vi "First model found in list.vi"(8 "Models to look for":string[](array[string])=["33120A", "33220A", "AFG2021"], 9 "Models IN":string[](array[string])) -> (2 "First Model Found":string, 3 "Models Passthrough":string[](array[string]))   [LabVIEW 2019]
doc: "Comapres the list of connected instruments to a sepcific list of devices of a certain class that the user is looking for.\n\"Models In\" is the Array of models returned by the \"Get Ports\" VI\n\"Models to Look For\" is an Array defined by the user. The array is a list of similar devices of a certain type. The first element of the array is the model needed for the procedure. The following elements are suitable substitutes.\n\"First Model Found\" is a STRING that is the Model matched in the connected devices array and the user defined array. \ni.e. 5522A, 5520A 5500A"
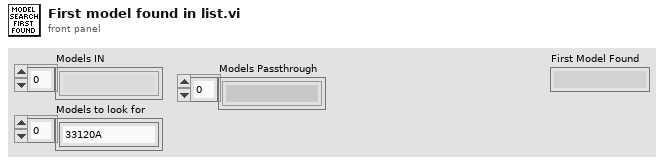
[diagram p1: front panel]
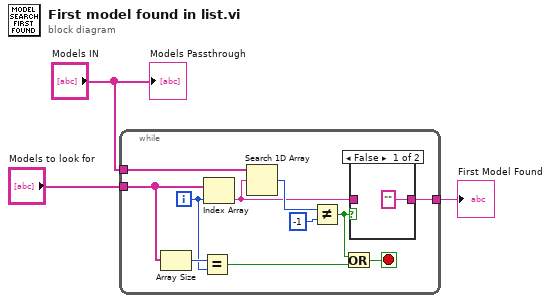
[diagram p0: block diagram]
diagram:
  n1 = while {
    tunnel: "Models to look for" -> [w12]
    tunnel: [w5] -> w1
    tunnel: "Models IN" -> [w4]
    i -> [w9]
    stop <- w11 stop-if-true
    n2 = Array Size(array=w12) -> (size(s)=w10:i32)
    n3 = Equal?(x=w10, y=w9) -> (x = y?=w8:bool)
    n4 = Index Array(array=w12, index=w9) -> (element=w6:string)
    n5 = Search 1D Array(1D array=w4, element=w6) -> (index of element=w14:i32)  [unwired: 1 in]
    n6 = Not Equal?(x=w14, y=-1) -> (x != y?=w7:bool)
    n7 = Or(x=w7, y=w8) -> (x .or. y?=w11:bool)
    n8 = case shown="False" w7 {
      tunnel: w6 -> [_ w16]
      tunnel: ["" w16] -> w5
      frame False {
      }
      frame True {
      }
    }
  }
  "First Model Found" <- w1
  "Models Passthrough" <- "Models IN"
